vi "countrate.vi"() -> ()   [LabVIEW 2015]
uses:
  <vilib>/Platform/TimedLoop/XDataNode/timing_clust.ctl
  <vilib>/Platform/TimedLoop/XDataNode/nitl_modes.ctl
  <vilib>/Platform/TimedLoop/XDataNode/wakeup.ctl
  <vilib>/imath/engines/lvmath2/RunTimeEngine/Managers/WorkSpace/UID Generator.vi
  <vilib>/imath/engines/lvmath2/RunTimeEngine/RunTimeType/NIMS_RunTimeType_From StrictType (excl LVString).vi
  <instcachedir>/0/NIMS_RunTimeType_From StrictType (excl LVString)_EB1C38A9BC5048DA9ABDA8F781E54D21.lvgen/NIMS_RunTimeType_From StrictType (excl LVString)_EB1C38A9BC5048DA9ABDA8F781E54D21_000.vi
  <vilib>/imath/engines/lvmath2/RunTimeEngine/RunTimeType/NIMS_RunTimeType_Set Source Original Bool.vi
  <vilib>/imath/engines/lvmath2/RunTimeEngine/LocalVariableDefStatement/MC_LocalVariableDefStatement_Display.vi
  <vilib>/imath/engines/lvmath2/RunTimeEngine/Managers/SymbolTable/Clear UID.vi
  <vilib>/imath/engines/lvmath2/RunTimeEngine/NodeEndStatement/NIMS_NodeEndStatement_Output.vi
  <instcachedir>/0/NIMS_NodeEndStatement_Output_53EC0D466D134D7ABD903AC30B43404B.lvgen/NIMS_NodeEndStatement_Output_53EC0D466D134D7ABD903AC30B43404B_013.vi
  <vilib>/imath/engines/lvmath2/RunTimeEngine/ErrorHandling/NIMS_Finalize Error.vi
  <vilib>/Utility/file.llb/Write Delimited Spreadsheet (I64).vi
  <vilib>/platform/TimedLoop/XDataNode/XDataNode.xnode
  <vilib>/Platform/TimedLoop/XDataNode/XDNodeRunTimeDep.lvlib
  <vilib>/imath/engines/lvmath2/RunTimeEngine/Managers/SymbolTable/NIMS_WorkSpace.lvlib
panel:
  in  "AquisitionTime":dbl
  in  "Period":dbl
  out "XY Graph":cluster{i32[], i32[]}(graph)
  out "counts per second":dbl(knob) scale=0.0..100.0
  # "Demo count rate VI for Physics 434"
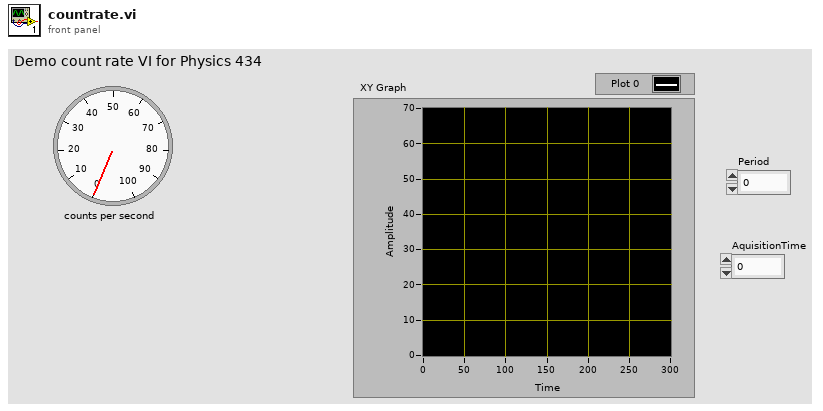
[diagram p1: front panel]
types:
  T1 = typedef "XDNodeRunTimeDep.lvlib/timing_clust.ctl" = cluster{"Expected End [f-1]":u64, "Actual End [f-1]":u64, "Finished Late? [f-1]":bool, "Expected End [i-1]":u64, "Actual End [i-1]":u64, "Finished Late? [i-1]":bool, "Expected Start [i]":u64, "Actual Start [i]":u64, "Expected Start [f]":u64, "Actual Start [f]":u64, "Source Name":string, "Structure Name":string, "Period":i64, "Deadline":i64, "Offset":i64, "Start":i64, "Priority":i32, "Timeout":i32, "Mode":T2, "Wakeup Reason":T3, "Error":errorcluster, "Source Type":string, "Secondary Source Type":string, "Global End Time":u64, "Global Start Time":u64, "Frame Duration":u64, "Iteration Duration":u64, "Assigned CPU":i32, "I/O Scan Engine Mode":u32}
  T2 = typedef "XDNodeRunTimeDep.lvlib/nitl_modes.ctl" = enum32{"No Change", "Process missed periods, maintain original phase", "Discard missed periods, maintain original phase", "Process missed periods, ignore original phase", "Discard missed periods, ignore original phase"}
  T3 = typedef "XDNodeRunTimeDep.lvlib/wakeup.ctl" = enum32{"Normal", "Aborted", "Asynchronous wakeup", "Timing source error", "Timed loop error", "Timeout"}
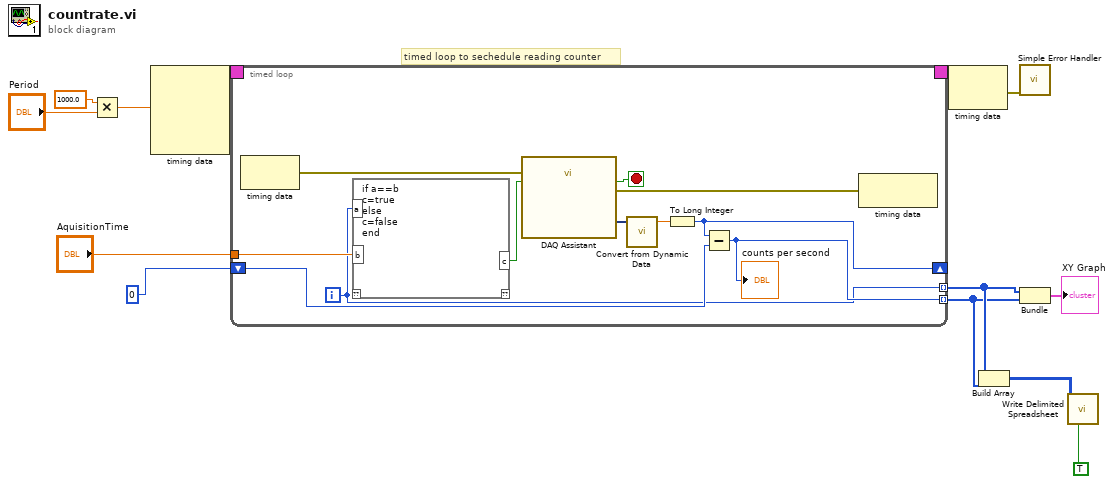
[diagram p0: block diagram]
diagram:
  # "timed loop to sechedule reading counter"
  n1 = Multiply(x=1000.0, y="Period") -> (x*y=w8:dbl)
  n2 = node-c288(w8) -> (w13:T1)  [unwired: 3 in]
  n3 = timed-loop {
    timing: w13 -> [_]
    timing-out: [_] -> w12
    shift-right: [w21] -> _
    shift-left: 0 -> [w23]
    tunnel: [w17] -> w4 mode=indexing
    tunnel: [w15] -> w5 mode=indexing
    tunnel: "AquisitionTime" -> [w16]
    i -> [w15]
    stop <- w22 stop-if-true
    n4 = node-c288() -> (w18:errorcluster)  [unwired: 1 in]
    n5 = mathscript code="if a==b\nc=true\nelse\nc=false\nend"("a"=w15, "b"=w16) -> ("c"=w14:bool)  [unwired: 1 in, 1 out]
    n6 = call "DAQ Assistant"("error in"=w18, "stop (F)"=w14) -> ("data"=w24:dynamicdata, "stopped"=w22:bool, "error out"=w19:errorcluster)  [unwired: 14 in, 1 out]
    n7 = call "Convert from Dynamic Data"("Dynamic Data Type"=w24) -> ("Scalar"=w20:dbl)  [unwired: 3 in]
    n8 = To Long Integer(number=w20) -> (32bit integer=w21:i32)
    n9 = Subtract(x=w21, y=w23) -> (x-y=w17:i32)
    "counts per second" <- w17
    n10 = node-c288(w19) -> ()  [unwired: 1 out]
  }
  n11 = node-c288(w12) -> (w10:errorcluster)
  n12 = Build Array(w5, w4) -> (w3:i32[][])
  n13 = call <vilib>:"Simple Error Handler.vi"("error in (no error)"=w10) -> ()  [unwired: 4 in, 5 out]
  n14 = Bundle(w5, w4) -> (→"XY Graph":cluster{i32[], i32[]})  [unwired: 1 in]
  n15 = call-poly <vilib>:"Write Delimited Spreadsheet.vi"("2D data"=w3, "transpose? (F)"=TRUE) -> ()  [unwired: 12 in, 2 out]
